vi "Corr_stats_labels.vi"(2 "Inst 2 Units":T1={"Colour"=0, "Inst type"=enum."Pitot-static tube", "Inst name"="Manometer voltage", "Symbol"="U", "Code name"="", "Extra Info"="U", "Inst Array"=enum."PWA", "Extra Titles"=[], "Extra Values"=[], "U"=0.0, "u^2"=0.0, "u^3"=0.0, "u^4"=0.0, "Skew_u"=0.0, "Kurt_u"=0.0, "Sd Error in Mean"=0.0, "% u'/U"=0.0, "X"=0.0, "Y"=0.0, "Z"=0.0, "Timescale integral Estimate"=0.0, "Sd Error in Variance"=0.0, "Calib File"=path "", "Calib Constants"=[], "Output Position"=FALSE, "Full Stats"=FALSE, "Av Sampling Rate"=0.0, "Av No of Samples"=0.0, "Total Meas Time (s)"=0.0, "ADAM Ch Name"="", "Max value"=0.0, "Min value"=0.0} {"Sd Error in Variance" format="%.2f"; "Skew_u" format="%.2f"; "% u'/U" format="%.2f"; "Sd Error in Mean" format="%.2f"; "Kurt_u" format="%.2f"; "u^4" format="%.2f"; "u^3" format="%.2f"; "U" format="%.2f"; "u^2" format="%.2f"}, 3 "Inst 1 Units":T1={"Colour"=0, "Inst type"=enum."Pitot-static tube", "Inst name"="Manometer voltage", "Symbol"="U", "Code name"="", "Extra Info"="U", "Inst Array"=enum."PWA", "Extra Titles"=[], "Extra Values"=[], "U"=0.0, "u^2"=0.0, "u^3"=0.0, "u^4"=0.0, "Skew_u"=0.0, "Kurt_u"=0.0, "Sd Error in Mean"=0.0, "% u'/U"=0.0, "X"=0.0, "Y"=0.0, "Z"=0.0, "Timescale integral Estimate"=0.0, "Sd Error in Variance"=0.0, "Calib File"=path "", "Calib Constants"=[], "Output Position"=FALSE, "Full Stats"=FALSE, "Av Sampling Rate"=0.0, "Av No of Samples"=0.0, "Total Meas Time (s)"=0.0, "ADAM Ch Name"="", "Max value"=0.0, "Min value"=0.0} {"Sd Error in Variance" format="%.2f"; "Skew_u" format="%.2f"; "% u'/U" format="%.2f"; "Sd Error in Mean" format="%.2f"; "Kurt_u" format="%.2f"; "u^4" format="%.2f"; "u^3" format="%.2f"; "U" format="%.2f"; "u^2" format="%.2f"}) -> (0 "Output":string[](array[string]))   [LabVIEW 2016]
uses:
  Controls/Analysis_info_cluster.ctl
  Controls/Inst_type.ctl
  Controls/Instrument_Array.ctl
  Globals/Meas_global.vi
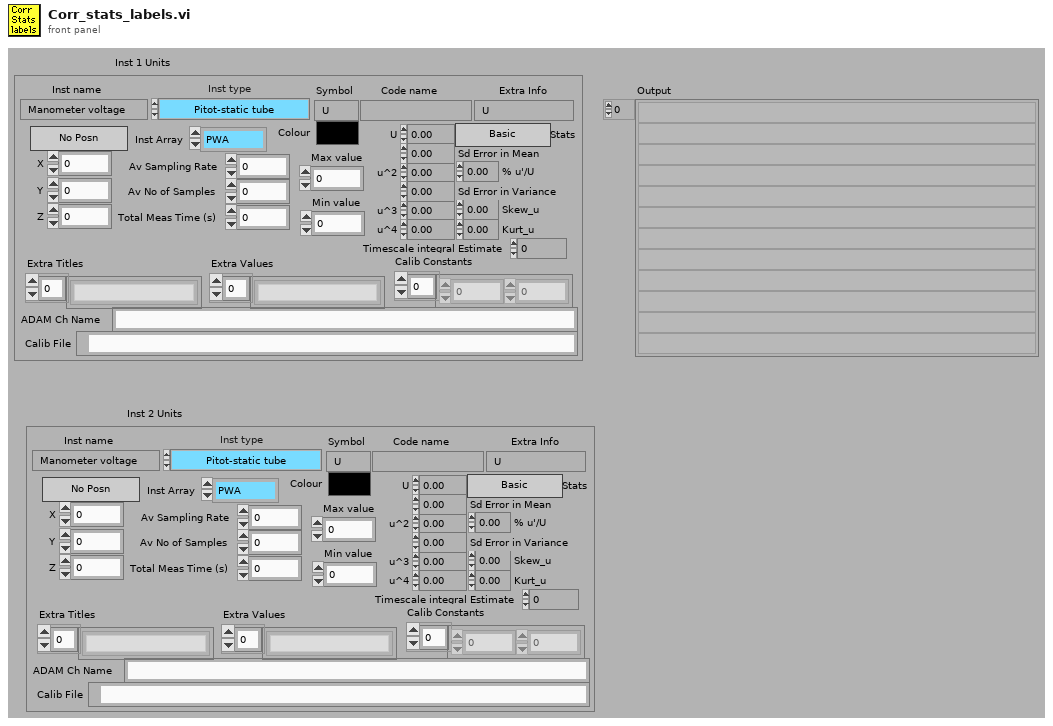
[diagram p1: front panel]
types:
  T1 = typedef "Analysis_info_cluster.ctl" = cluster{"Colour":u32, "Inst type":T2, "Inst name":string, "Symbol":string, "Code name":string, "Extra Info":string, "Inst Array":T3, "Extra Titles":string[], "Extra Values":string[], "U":dbl, "u^2":dbl, "u^3":dbl, "u^4":dbl, "Skew_u":dbl, "Kurt_u":dbl, "Sd Error in Mean":dbl, "% u'/U":dbl, "X":dbl, "Y":dbl, "Z":dbl, "Timescale integral Estimate":dbl, "Sd Error in Variance":dbl, "Calib File":path, "Calib Constants":dbl[], "Output Position":bool, "Full Stats":bool, "Av Sampling Rate":dbl, "Av No of Samples":dbl, "Total Meas Time (s)":dbl, "ADAM Ch Name":string, "Max value":dbl, "Min value":dbl}
  T2 = typedef "Inst_type.ctl" = enum16{"Propeller anemometer", "Raw voltage", "Pressure Transducer", "Pitot-static tube", "Preston tube", "Hot wire", "Cross wire 1", "Cross wire 2", "Generic Linear", "Generic Polynomial", "Generic BackPoly", "Fast FID", "Thermocouple", "Cold wire", "Pulsed Wire", "LDA Vel", "LDA Tran time", "LDA Arr time", "Microphone"}
  T3 = typedef "Instrument_Array.ctl" = enum16{"PWA", "LDA", "Analogue"}
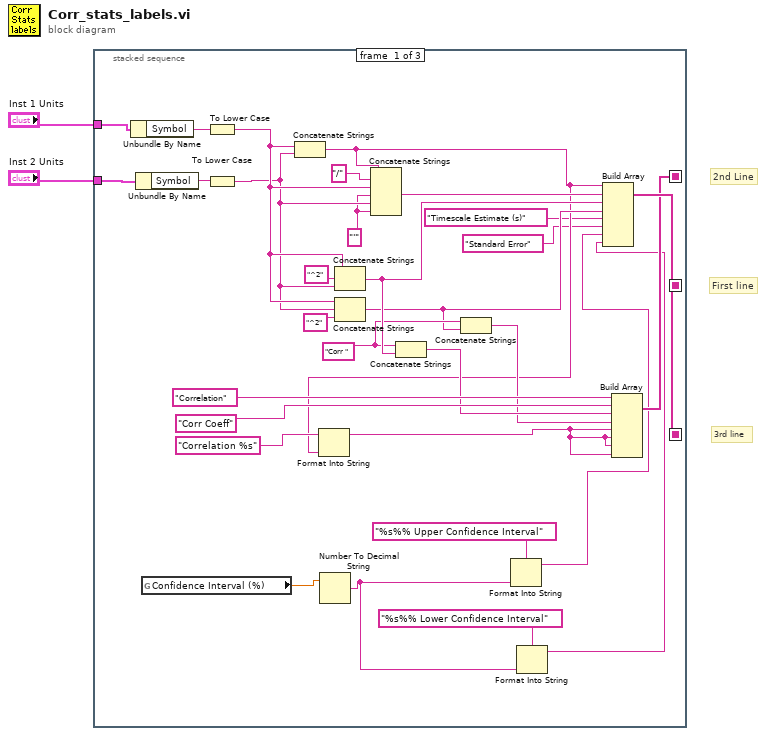
[diagram p0: block diagram]
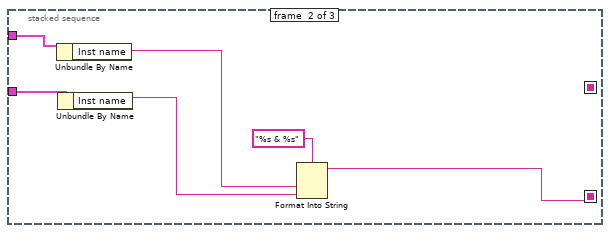
[diagram p2: hidden frame]
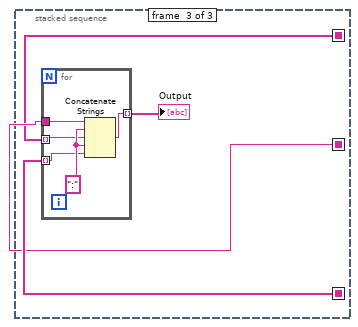
[diagram p3: hidden frame]
diagram:
  # "First line"
  # "2nd Line"
  # "3rd line"
  n1 = stacked-sequence {
    seq-local: [w25 _ _] -> [_ _ w43]
    seq-local: [w24 _ _] -> [_ _ w40]
    seq-local: [_ w34 _] -> [_ _ w41]
    tunnel: "Inst 2 Units" -> [w29 w38 _]
    tunnel: "Inst 1 Units" -> [w26 w39 _]
    frame #0 {
      w16 = "Corr "
      w20 = "'"
      n2 = Unbundle By Name(w26) -> ("Symbol"=w28:string)
      n3 = Unbundle By Name(w29) -> ("Symbol"=w27:string)
      n4 = global read "Meas_global.vi" "Confidence Interval (%)"() -> (w12:dbl)
      n5 = To Lower Case(string=w28) -> (all lower case string=w33:string)
      n6 = To Lower Case(string=w27) -> (all lower case string=w32:string)
      n7 = Concatenate Strings(w33, w32) -> (w10:string)
      n8 = Format Into String(format string="Correlation %s", w10) -> (resulting string=w9:string)  [unwired: 2 in, 1 out]
      n9 = Number To Decimal String(number=w12) -> (decimal integer string=w7:string)  [unwired: 1 in]
      n10 = Concatenate Strings(w33, "^2", w32) -> (w18:string)
      n11 = Concatenate Strings(w33, w32, "^2") -> (w15:string)
      n12 = Concatenate Strings(w10, "/", w33, w20, w32, w20) -> (w19:string)
      n13 = Concatenate Strings(w16, w18) -> (w17:string)
      n14 = Concatenate Strings(w16, w15) -> (w14:string)
      n15 = Format Into String(format string="%s%% Upper Confidence Interval", w7) -> (resulting string=w6:string)  [unwired: 2 in, 1 out]
      n16 = Format Into String(format string="%s%% Lower Confidence Interval", w7) -> (resulting string=w5:string)  [unwired: 2 in, 1 out]
      n17 = Build Array(w10, w19, w18, w15, "Timescale Estimate (s)", "Standard Error", w6, w5) -> (w25:string[])
      n18 = Build Array("Correlation", "Corr Coeff", w17, w14, w9, w9, w9, w9) -> (w24:string[])
    }
    frame #1 {
      n19 = Unbundle By Name(w39) -> ("Inst name"=w36:string)
      n20 = Unbundle By Name(w38) -> ("Inst name"=w35:string)
      n21 = Format Into String(format string="%s & %s" ("Format String"), w36, w35) -> (resulting string=w34:string)  [unwired: 2 in, 1 out]
    }
    frame #2 {
      n22 = for {
        tunnel: [w48] -> w42 mode=indexing
        tunnel: w41 -> [w47]
        tunnel: w40 -> [w45] mode=indexing
        tunnel: w43 -> [w44] mode=indexing
        w46 = ":" ("Substring")
        n23 = Concatenate Strings(w47, w46, w45, w46, w44) -> (w48:string)
      }
      "Output" <- w42
    }
  }
